vi "String to Boolean.vi"(11 "Bool String":string) -> (3 "Boolean":bool)   [LabVIEW 2018, in "JSON.lvlib"]
uses:
  JSON.lvlib
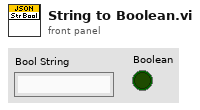
[diagram p1: front panel]
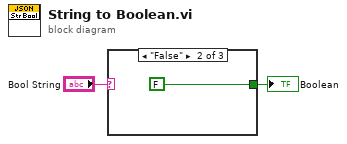
[diagram p0: block diagram]
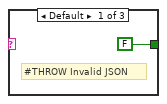
[diagram p2: hidden frame]
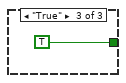
[diagram p3: hidden frame]
diagram:
  n1 = case shown="\"False\"" "Bool String" {
    tunnel: [FALSE FALSE TRUE] -> w1
    frame Default {
      # "#THROW Invalid JSON"
    }
    frame "False" {
    }
    frame "True" {
    }
  }
  "Boolean" <- w1
